vi "0.vi"(11 "文字列入力":string) -> (3 "文字列出力":string)   [LabVIEW 2019]
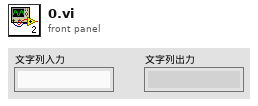
[diagram p1: front panel]
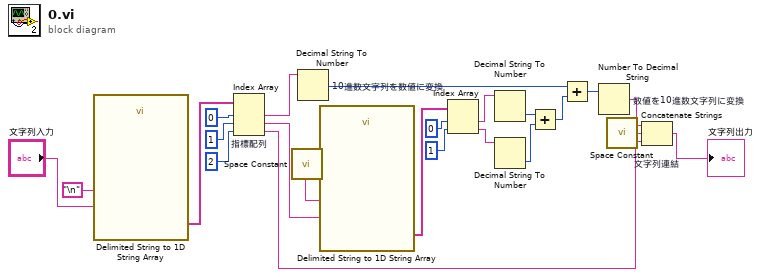
[diagram p0: block diagram]
diagram:
  n1 = call <vilib>:"Delimited String to 1D String Array.vi"("delimiter"="\n", "delimited string"="文字列入力") -> ("string array"=w2:string[])  [unwired: 9 in]
  n2 = Index Array "指標配列"(array=w2, index #1=0, index #2=1, index #3=2) -> (element #1=w7:string, element #2=w8:string, element #3=w22:string)
  n3 = call <vilib>:"Space Constant.vi"() -> ("String"=w9:string)
  n4 = Decimal String To Number "10進数文字列を数値に変換"(string=w7) -> (number=w16:i32)  [unwired: 2 in, 1 out]
  n5 = call <vilib>:"Delimited String to 1D String Array.vi"("delimiter"=w9, "delimited string"=w8) -> ("string array"=w10:string[])  [unwired: 9 in]
  n6 = Index Array(array=w10, index #1=0, index #2=1) -> (element #1=w13:string, element #2=w14:string)
  n7 = Decimal String To Number(string=w13) -> (number=w17:i32)  [unwired: 2 in, 1 out]
  n8 = Decimal String To Number(string=w14) -> (number=w18:i32)  [unwired: 2 in, 1 out]
  n9 = Add(x=w17, y=w18) -> (x+y=w15:i32)
  n10 = Add(x=w16, y=w15) -> (x+y=w19:i32)
  n11 = Number To Decimal String "数値を10進数文字列に変換"(number=w19) -> (decimal integer string=w20:string)  [unwired: 1 in]
  n12 = call <vilib>:"Space Constant.vi"() -> ("String"=w21:string)
  n13 = Concatenate Strings "文字列連結"(w20, w21, w22) -> (→"文字列出力":string)
